vi "GetJoystickAxes.vi"(9 "Axes ID":dbl, 11 "JoystickDevRef":T1) -> (2 "element":dbl)   [LabVIEW 2014]
doc: "Gets one of the Axes from the joystick."
uses:
  <vilib>/Rock Robotics/WPI/Joystick/WPI_JoystickDevRef.ctl
  <vilib>/Rock Robotics/WPI/Joystick/WPI_JoystickDeviceEnum.ctl
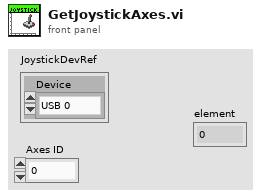
[diagram p1: front panel]
types:
  T1 = typedef "WPI_JoystickDevRef.ctl" = cluster{"Device":T2}
  T2 = typedef "WPI_JoystickDeviceEnum.ctl" = enum16{"USB 0", "USB 1", "USB 2", "USB 3", "USB 4", "USB 5"}
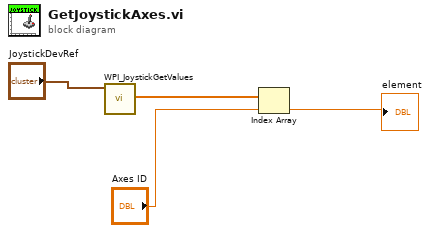
[diagram p0: block diagram]
diagram:
  n1 = call <vilib>:"WPI_JoystickGetValues.vi"("JoystickDevRef"="JoystickDevRef") -> ("Axes"=w3:dbl[])  [unwired: 6 in, 4 out]
  n2 = Index Array(array=w3, index="Axes ID") -> (element=→"element":dbl)
